vi "Build Raw Parameter Data.vi"(8 "error in (no error)":errorcluster, 10 "FPGA Data":u16[](array[numeric]), 11 "Async Message in":refnum<class "Async Message.lvclass">) -> (0 "error out":errorcluster, 1 "Parameter Data":u64[](array[numeric]), 2 "Parameters":string[](array[string]), 3 "Async Message out":refnum<class "Async Message.lvclass">)   [LabVIEW 2020, in "BCI-1553 API.lvlib" / "Async Message.lvclass"]
doc: "<DO NOT CALL>\n\nParses out the base word and 3 additional data values to attempt to get the entire possible raw parameter data word."
uses:
  Async Message.lvclass
  Async Message.lvclass/Async Message.ctl
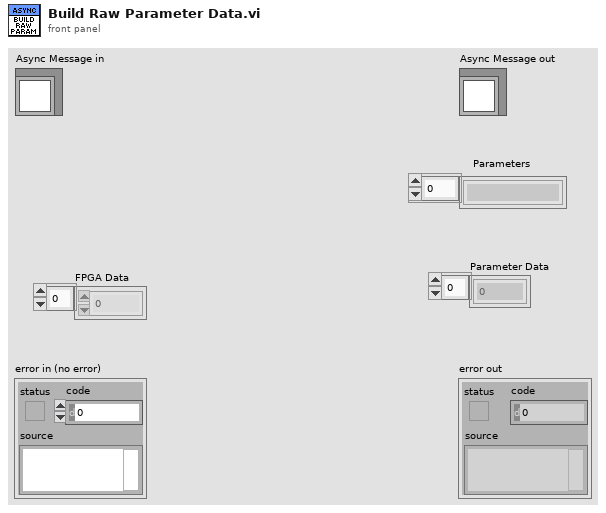
[diagram p1: front panel]
types:
  T1 = typedef "BCI-1553 API.lvlib/Parameter Table Data.ctl" = cluster{"Parameter Name":string, "Base Word":u16, "Address":u16, "Value":u64, "Mask":u16[], "Scaling Info":T2}
  T2 = typedef "BCI-1553 API.lvlib/Scaling Information.ctl" = cluster{"Bit Offset":i32, "Bit Count":i32, "LSB Resolution":dbl, "2's Complement":bool, "Big Endian":bool, "Sign Bit":bool}
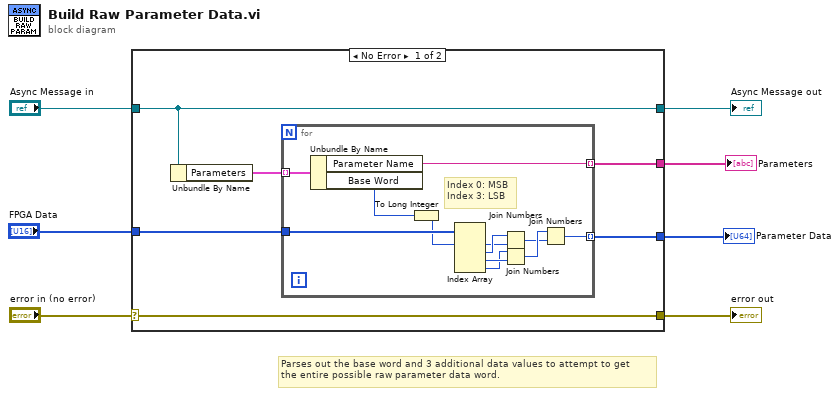
[diagram p0: block diagram]
diagram:
  # "Parses out the base word and 3 additional data values to attempt to get\nthe entire possible raw parameter data word."
  n1 = case shown="No Error" "error in (no error)" {
    selector: "error in (no error)" -> [w13 w27]
    tunnel: [w13 w27] -> w6
    tunnel: [w12 w26] -> w4
    tunnel: "Async Message in" -> [w12 w26]
    tunnel: "FPGA Data" -> [w11 _]
    tunnel: [w9 _] -> w2
    tunnel: [w8 _] -> w1
    frame No Error {
      n2 = Unbundle By Name(w12) -> ("Parameters"=w10:T1[])
      n3 = for {
        tunnel: w11 -> [w19]
        tunnel: w10 -> [w25] mode=indexing
        tunnel: [w16] -> w9 mode=indexing
        tunnel: [w15] -> w8 mode=indexing
        # "Index 0: MSB\nIndex 3: LSB"
        n4 = Unbundle By Name(w25) -> ("Parameter Name"=w15:string, "Base Word"=w14:u16)
        n5 = To Long Integer(number=w14) -> (32bit integer=w18:i32)
        n6 = Index Array(array=w19, index #1=w18) -> (element #1=w21:u16, element #2=w22:u16, element #3=w20:u16, element #4=w17:u16)  [unwired: 3 in]
        n7 = Join Numbers(hi=w22, lo=w21) -> ((hi.lo)=w23:u32)
        n8 = Join Numbers(hi=w17, lo=w20) -> ((hi.lo)=w24:u32)
        n9 = Join Numbers(hi=w24, lo=w23) -> ((hi.lo)=w16:u64)
      }
    }
    frame Error {
    }
  }
  "error out" <- w6
  "Async Message out" <- w4
  "Parameter Data" <- w2
  "Parameters" <- w1
